vi "Find Matching Descriptions.vi"(8 "error in":errorcluster, 10 "File ID":i32, 11 "Peer Review in":refnum<class "Peer Review.lvclass">) -> (0 "error out":errorcluster, 3 "Peer Review out":refnum<class "Peer Review.lvclass">)   [LabVIEW 2020, in "Peer Review.lvclass"]
uses:
  Peer Review.lvclass
  Peer Review.lvclass/Peer Review.ctl
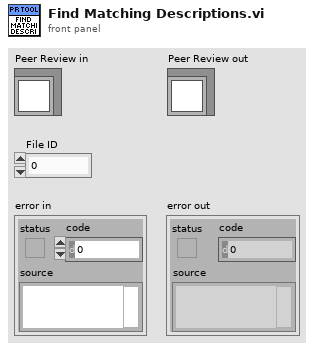
[diagram p1: front panel]
types:
  T1 = typedef "Peer Review.lvclass/File Info.ctl" = cluster{"File ID":i32, "Commit ID":i32, "Reviewed Hash":string, "Relative Path":string, "File Path":path, "File Checksum":string, "State":T2, "FP Changes":i32, "BD Changes":i32, "FP Bounds Error":dbl, "BD Bounds Error":dbl, "Lines Added":i32, "Lines Removed":i32, "Analysis Passes":i32, "Analysis Fails":i32, "Attribute Changes":i32, "Reentrancy Changes":string, "Cyclomatic Complexity":i32, "Node Count":u32, "Revision Number":u32, "LabVIEW Version":string, "Description":string, "Master Path":path, "Master Checksum":string, "VI Type":T3, "LabVIEW File":bool, "Review Complete":bool, "File Ref":refnum<vi>}
  T2 = typedef "Peer Review.lvclass/File State.ctl" = enum16{"Interrogation Needed", "Modified", "Deleted", "Added", "Matches Previous", "No Changes", "Moved"}
  T3 = typedef "Peer Review.lvclass/VI Type.ctl" = enum32{"invalid VI type", "Standard VI", "Control VI", "Global VI", "Polymorphic VI", "Configuration VI", "SubSystem", "Facade VI", "Method VI", "Statechart Diagram VI"}
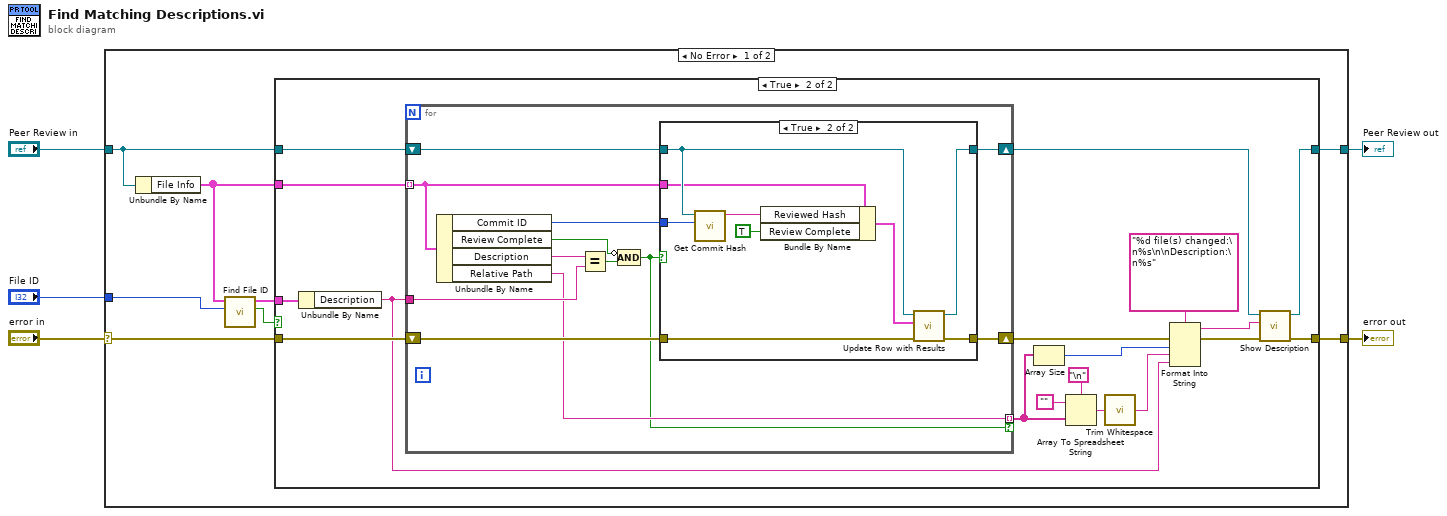
[diagram p0: block diagram]
diagram:
  n1 = case shown="No Error" "error in" {
    selector: "error in" -> [w12 w58]
    tunnel: "File ID" -> [w13 _]
    tunnel: [w7 w58] -> w3
    tunnel: "Peer Review in" -> [w9 w57]
    tunnel: [w6 w57] -> w1
    frame No Error {
      n2 = Unbundle By Name(w9) -> ("File Info"=w10:T1[])
      n3 = call "Find File ID.vi"("File ID"=w13, "File List"=w10) -> ("Found?"=w8:bool, "File Info"=w11:T1)  [unwired: 7 in, 1 out]
      n4 = case shown="True" w8 {
        tunnel: w12 -> [w14 w33]
        tunnel: w11 -> [_ w32]
        tunnel: w10 -> [_ w31]
        tunnel: w9 -> [w15 w30]
        tunnel: [w15 w18] -> w6
        tunnel: [w14 w17] -> w7
        frame False {
        }
        frame True {
          n5 = Unbundle By Name(w32) -> ("Description"=w16:string)
          n6 = for {
            tunnel: w31 -> [w44] mode=indexing
            tunnel: w16 -> [w45]
            shift-right: [w41] -> w27
            shift-left: w33 -> [w43]
            shift-right: [w40] -> w19
            shift-left: w30 -> [w42]
            tunnel: [w35] -> w26 mode=indexing if=w34
            n7 = Unbundle By Name(w44) -> ("Commit ID"=w39:i32, "Review Complete"=w36:bool, "Description"=w38:string, "Relative Path"=w35:string)
            n8 = Equal?(x=w38, y=w45) -> (x = y?=w37:bool)
            n9 = Compound Arithmetic op=AND(invert w36, w37) -> (w34:bool)
            n10 = case shown="True" w34 {
              tunnel: w44 -> [_ w48]
              tunnel: w43 -> [w46 w55]
              tunnel: w42 -> [w47 w51]
              tunnel: [w46 w53] -> w41
              tunnel: [w47 w52] -> w40
              tunnel: w39 -> [_ w50]
              frame False {
              }
              frame True {
                n11 = call "Get Commit Hash.vi"("Commit ID"=w50, "Peer Review"=w51) -> ("Hash"=w49:string)  [unwired: 9 in]
                n12 = Bundle By Name(cluster=w48, "Reviewed Hash"=w49, "Review Complete"=TRUE ("Review Complete?")) -> (w54:T1)
                n13 = call "Update Row with Results.vi"("error in"=w55, "File Info"=w54, "Peer Review in"=w51) -> ("error out"=w53:errorcluster, "Peer Review out"=w52:refnum<class "Peer Review.lvclass">)  [unwired: 7 in]
              }
            }
          }
          n14 = Array Size(array=w26) -> (size(s)=w25:i32)
          n15 = Array To Spreadsheet String(delimiter (Tab)="\n", array=w26, 3:"") -> (spreadsheet string=w24:string)
          n16 = call <vilib>:"Trim Whitespace.vi"("string"=w24) -> ("trimmed string"=w23:string)  [unwired: 1 in]
          n17 = Format Into String(format string="%d file(s) changed:\n%s\n\nDescription:\n%s", error in=w27, w25, w23, w16) -> (resulting string=w20:string, error out=w21:errorcluster)  [unwired: 1 in]
          n18 = call "Show Description.vi"("error in"=w21, "Description"=w20, "Peer Review in"=w19) -> ("error out"=w17:errorcluster, "Peer Review out"=w18:refnum<class "Peer Review.lvclass">)  [unwired: 7 in]
        }
      }
    }
    frame Error {
    }
  }
  "error out" <- w3
  "Peer Review out" <- w1
